vi "Liquefaction Detection.vi"() -> ()   [LabVIEW 2023]
doc: "This example shows the application of the Time Frequency Analysis VIs in seismic engineering. \n\nThe strength and stiffness of the soil might be impaired when an earthquake occurs. This phenomenon is called liquefaction. The horizontal ground motions can indicate whether there is liquefaction. The frequency of the horizontal acceleration decreases if there is liquefaction in the soil. The mean instantaneous frequency (MIF) estimated from the time-frequency representation of the horizontal acceleration signal can be used to detect the existence of liquefaction. The MIF value drops below 1 Hz when there is liquefaction.\n\nThis example uses the TFA Gabor Spectrogram VI to compute the time-frequency representation of the signals and then uses the TFA Mean Instantaneous Frequency VI to compute the MIF values of the signals.\n\n<b>Instructions:</b>\n1) Run this VI.\n2) Observe the difference in frequency values between the MIF of liquefaction and the MIF of a liquefaction-free signal."
uses:
  <vilib>/addons/Time Frequency Analysis/typedefs.llb/TFA Data.ctl
  <vilib>/addons/Time Frequency Analysis/Spectrogram.llb/TFA Fast Gabor Spectrogram (Waveform).vi
  <vilib>/addons/Time Frequency Analysis/_control.llb/TFA Configure Spectrogram Indicator (Predefined Color Table).vi
  <vilib>/addons/_Advanced Signal Processing/NI_AdvSigProcTFA.lvlib
panel:
  out "aspt-left-top":bool
  out "Spectrogram_Free":dbl[][](graph) caption="Spectrogram"
  out "Spectrogram":dbl[][](graph)
  out "Mean Instantaneous_Free Frequency":cluster{"t0":dbl, "dt":dbl, "frequency":dbl[]}(graph) caption="Mean Instantaneous Frequency"
  out "Mean Instantaneous Frequency":cluster{"t0":dbl, "dt":dbl, "frequency":dbl[]}(graph)
  out "Time Domain Signal_Free":waveform(dbl)(graph) caption="Time Domain Signal"
  out "Time Domain Signal":waveform(dbl)(graph)
  # "Overview: Shows the application of the Time Frequency Analysis VIs in seismic engineering.\nRequirements: LabVIEW Full Development System, Advanced Signal Processing Toolkit\nInstructions: \n1. Run this VI.\n2. Observe the difference in frequency values between the MIF of liquefaction and the MIF of a liquefaction-free signal."
  # "Liquefaction (Has Earthquake)"
  # "Liquefaction Free (No Earthquake)"
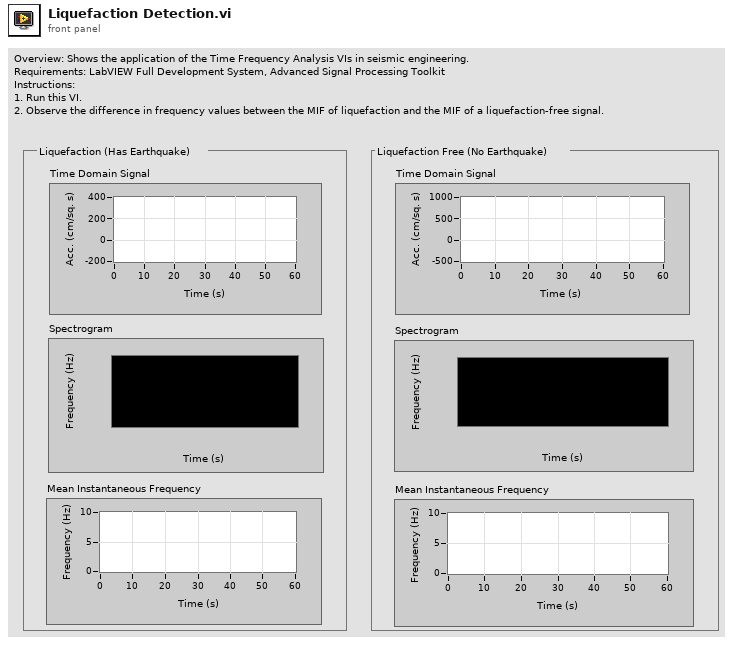
[diagram p1: front panel]
types:
  T1 = typedef "NI_AdvSigProcTFA.lvlib/TFA Data.ctl" = u16
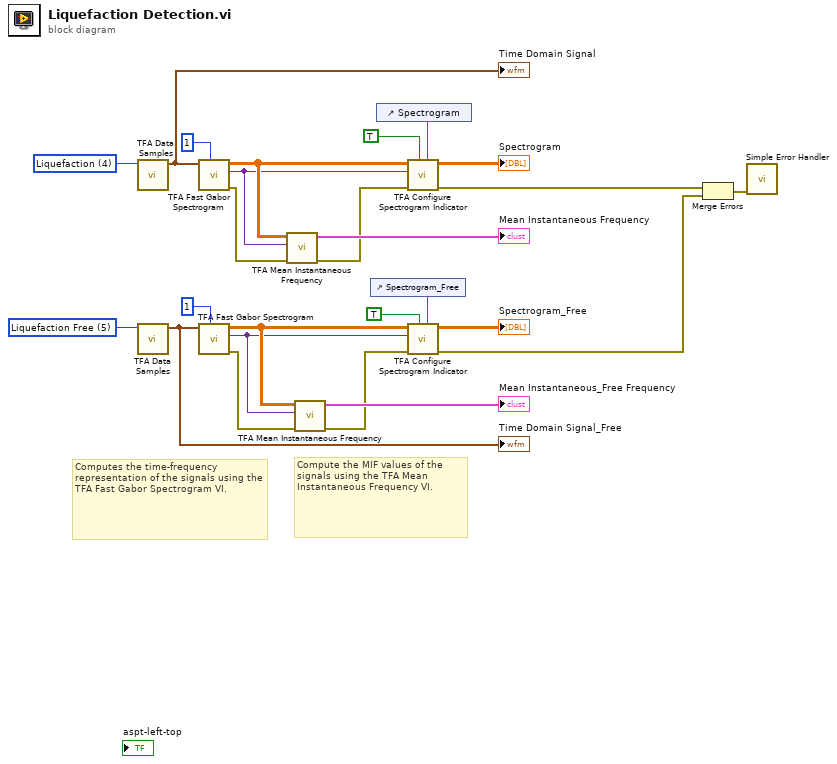
[diagram p0: block diagram]
diagram:
  w4 = T1 5 items=["PC Fan"=0, "Noisy Chirps"=1, "TDR 1"=2, "TDR 2"=3, "Liquefaction"=4, "Liquefaction Free"=5, "Aneurysm"=6, "Bat"=7, "RF"=8, "Two Gaussian"=9, "Three Gaussian"=10, "Chirp"=11, "Gaussian Chirp"=12, "Cross Chirp"=13, "Doppler"=14, "HOP"=15, "TF Sine"=16, "Three Tone"=17, "Four Tone"=23, "Blood Flow Doppler (phase a)"=20, "Blood Flow Doppler (phase b)"=21, "Heart sound"=22, "-"=18, "Random Noise"=19] ("data")
  w5 = T1 4 items=["PC Fan"=0, "Noisy Chirps"=1, "TDR 1"=2, "TDR 2"=3, "Liquefaction"=4, "Liquefaction Free"=5, "Aneurysm"=6, "Bat"=7, "RF"=8, "Two Gaussian"=9, "Three Gaussian"=10, "Chirp"=11, "Gaussian Chirp"=12, "Cross Chirp"=13, "Doppler"=14, "HOP"=15, "TF Sine"=16, "Three Tone"=17, "Four Tone"=23, "Blood Flow Doppler (phase a)"=20, "Blood Flow Doppler (phase b)"=21, "Heart sound"=22, "-"=18, "Random Noise"=19] ("data")
  # "Compute the MIF values of the signals using the TFA Mean Instantaneous Frequency VI."
  # "Computes the time-frequency representation of the signals using the TFA Fast Gabor Spectrogram VI."
  n1 = call <vilib>:"TFA Data Samples.vi"("data"=w5) -> ("signal"=w25:waveform(dbl))  [unwired: 10 out]
  "Time Domain Signal" <- w25
  n2 = call <vilib>:"TFA Data Samples.vi"("data"=w4) -> ("signal"=w24:waveform(dbl))  [unwired: 10 out]
  "Time Domain Signal_Free" <- w24
  n3 = call-poly <vilib>:"TFA Fast Gabor Spectrogram.vi"("order"=1, "signal"=w25) -> ("error out"=w21:errorcluster, "scale info"=w18:variant, "spectrogram"=w19:dbl[][])  [unwired: 3 in, 4 out]
  n4 = call-poly <vilib>:"TFA Fast Gabor Spectrogram.vi"("order"=1, "signal"=w24) -> ("error out"=w20:errorcluster, "scale info"=w12:variant, "spectrogram"=w13:dbl[][])  [unwired: 3 in, 4 out]
  n5 = call <vilib>:"TFA Mean Instantaneous Frequency.vi"("error in (no error)"=w21, "scale info"=w18, "spectrogram"=w19) -> ("error out"=w17:errorcluster, "MIF"=→"Mean Instantaneous Frequency":cluster{"t0":dbl, "dt":dbl, "frequency":dbl[]})  [unwired: 7 out]
  n6 = call <vilib>:"TFA Mean Instantaneous Frequency.vi"("error in (no error)"=w20, "scale info"=w12, "spectrogram"=w13) -> ("error out"=w11:errorcluster, "MIF"=→"Mean Instantaneous_Free Frequency":cluster{"t0":dbl, "dt":dbl, "frequency":dbl[]})  [unwired: 7 out]
  n7 = control-ref of="Spectrogram_Free"() -> (w9:refnum<vi>)
  n8 = control-ref of="Spectrogram"() -> (w14:refnum<vi>)
  n9 = call-poly <vilib>:"TFA Configure Spectrogram Indicator.vi"("reference of TF spectrogram indicator"=w14, "dB on? (F)"=TRUE ("dB"), "error in (no error)"=w17, "scale info"=w18, "spectrogram"=w19) -> ("error out"=w3:errorcluster, "TF spectrogram indicator"=→"Spectrogram":dbl[][])  [unwired: 2 in, 3 out]
  n10 = call-poly <vilib>:"TFA Configure Spectrogram Indicator.vi"("reference of TF spectrogram indicator"=w9, "dB on? (F)"=TRUE ("dB"), "error in (no error)"=w11, "scale info"=w12, "spectrogram"=w13) -> ("error out"=w2:errorcluster, "TF spectrogram indicator"=→"Spectrogram_Free":dbl[][])  [unwired: 2 in, 3 out]
  n11 = Merge Errors(w3, w2) -> (w1:errorcluster)
  n12 = call <vilib>:"Simple Error Handler.vi"("error in (no error)"=w1) -> ()  [unwired: 1 in, 8 out]
